vi "add_CMDInput.vi"(6 "Input":T1, 7 "msg in":string) -> (3 "msg out":string)   [LabVIEW 2018]
doc: "Flattens a pose 2D into a message"
uses:
  <userlib>/ROS for LabVIEW Software/ROS/MessageBuilding/std_msgs/subs/float64Scalar.vi
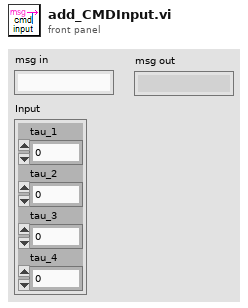
[diagram p1: front panel]
types:
  T1 = cluster{"tau_1":dbl, "tau_2":dbl, "tau_3":dbl, "tau_4":dbl}
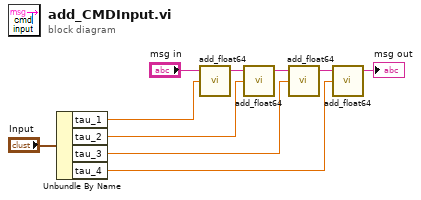
[diagram p0: block diagram]
diagram:
  n1 = Unbundle By Name("Input") -> ("tau_1"=w5:dbl, "tau_2"=w4:dbl, "tau_3"=w3:dbl, "tau_4"=w2:dbl)
  n2 = call-poly <userlib>:"add_float64.vi"("Numeric"=w5, "msg in"="msg in") -> ("msg out"=w8:string)  [unwired: 3 in]
  n3 = call-poly <userlib>:"add_float64.vi"("Numeric"=w4, "msg in"=w8) -> ("msg out"=w7:string)  [unwired: 3 in]
  n4 = call-poly <userlib>:"add_float64.vi"("Numeric"=w3, "msg in"=w7) -> ("msg out"=w6:string)  [unwired: 3 in]
  n5 = call-poly <userlib>:"add_float64.vi"("Numeric"=w2, "msg in"=w6) -> ("msg out"=→"msg out":string)  [unwired: 3 in]
